vi "Configure Measurement (Power Meter).vi"(0 "VISA resource name":refnum<visa-resource-name>, 1 "Video Bandwidth Type (0: High)":i32(ring) items=["High", "Medium", "Low", "Off"], 2 "Gate Start Time (0 seconds)":dbl, 5 "Auto Power Range Enable (T: Enable)":bool=TRUE, 7 "Power Range (0: Upper)":i32(ring) items=["Upper", "Lower"], 9 "Center Frequency (1000 Hz)":dbl=1000.0, 11 "error in (no error)":errorcluster, 12 "Interval Time (0.1 seconds)":dbl=0.1, 13 "Gate Measurement Type (0: Peak)":i32(ring) items=["Peak", "Peak to Average", "Average", "Minimum"]) -> (4 "VISA resource name out":refnum<visa-resource-name>, 15 "error out":errorcluster)   [LabVIEW 2022 SP3, in "Agilent N934X Series.lvlib"]
doc: "Configures the cable setting of Power Meter Option.\n\nNotes:\n(1) Option PWM or PWP is required to enable this function. Option PWM supports Keysight (Agilent) U2000 series USB average power sensor, and Option PWP supports Keysight (Agilent) U2020 X series peak power sensor.\n\n(2) This VI is only applicable for N9321C, N9322C, N9323C, N9324C models"
uses:
  <instrlib>/Agilent N934X Series/Agilent N934X Series.lvlib
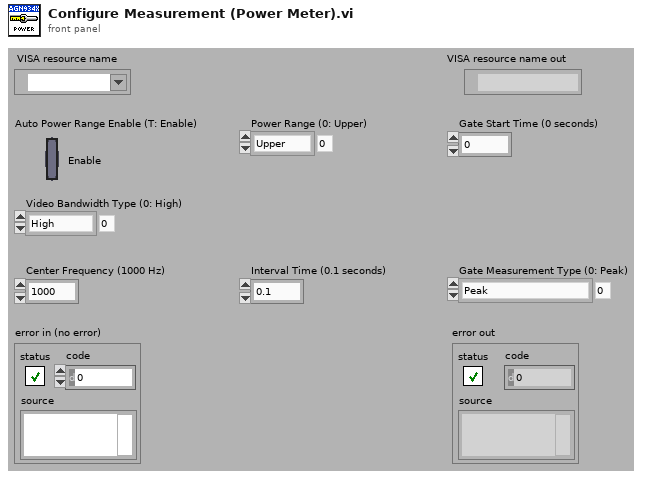
[diagram p1: front panel]
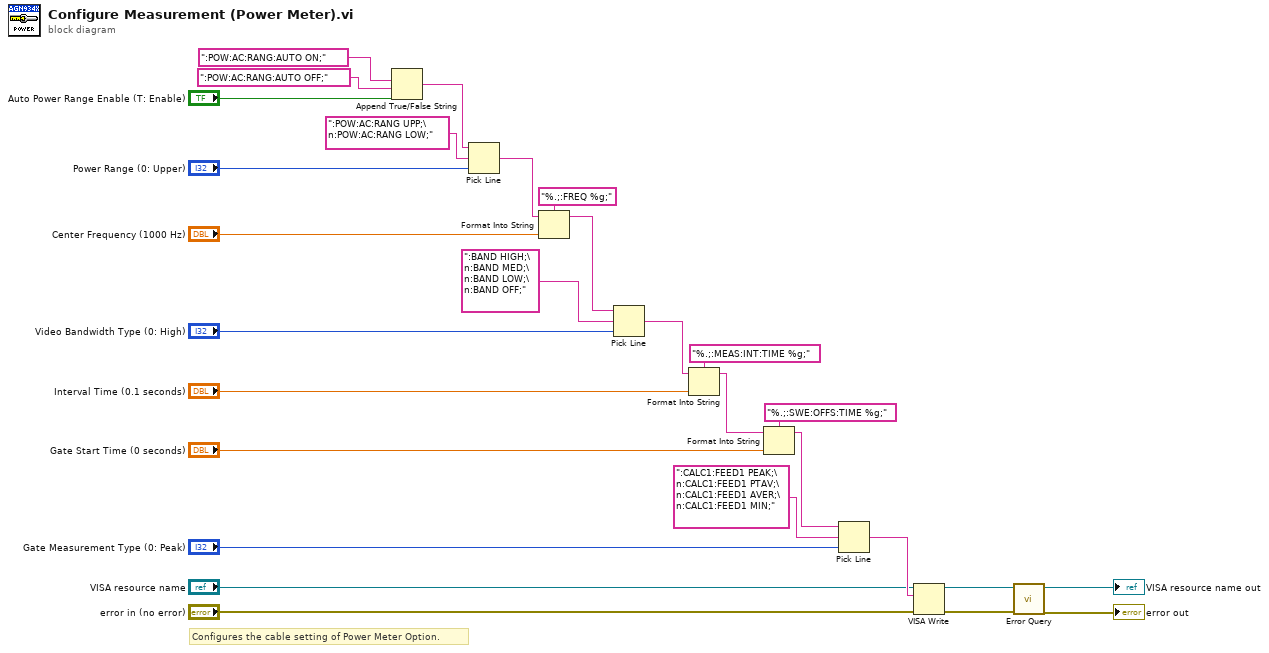
[diagram p0: block diagram]
diagram:
  # "Configures the cable setting of Power Meter Option."
  n1 = Append True/False String(1:"Auto Power Range Enable (T: Enable)", 2:":POW:AC:RANG:AUTO OFF;", 3:":POW:AC:RANG:AUTO ON;") -> (0:w1:string)  [unwired: 1 in]
  n2 = Pick Line(string ("")=w1, multi-line string=":POW:AC:RANG UPP;\n:POW:AC:RANG LOW;", line index="Power Range (0: Upper)") -> (output string=w2:string)
  n3 = Format Into String(format string="%.;:FREQ %g;", initial string=w2, "Center Frequency (1000 Hz)") -> (resulting string=w19:string)  [unwired: 1 in, 1 out]
  n4 = Pick Line(string ("")=w19, multi-line string=":BAND HIGH;\n:BAND MED;\n:BAND LOW;\n:BAND OFF;", line index="Video Bandwidth Type (0: High)") -> (output string=w18:string)
  n5 = Format Into String(format string="%.;:MEAS:INT:TIME %g;", initial string=w18, "Interval Time (0.1 seconds)") -> (resulting string=w15:string)  [unwired: 1 in, 1 out]
  n6 = Format Into String(format string="%.;:SWE:OFFS:TIME %g;", initial string=w15, "Gate Start Time (0 seconds)") -> (resulting string=w10:string)  [unwired: 1 in, 1 out]
  n7 = Pick Line(string ("")=w10, multi-line string=":CALC1:FEED1 PEAK;\n:CALC1:FEED1 PTAV;\n:CALC1:FEED1 AVER;\n:CALC1:FEED1 MIN;", line index="Gate Measurement Type (0: Peak)") -> (output string=w9:string)
  n8 = VISA Write(VISA resource name="VISA resource name", write buffer=w9, error in (no error)="error in (no error)") -> (VISA resource name out=w6:refnum<visa-resource-name>, error out=w5:errorcluster)  [unwired: 1 out]
  n9 = call <instrlib>:"Error Query.vi"("error in (no error)"=w5, "VISA resource name"=w6) -> ("error out"=→"error out":errorcluster, "VISA resource name out"=→"VISA resource name out":refnum<visa-resource-name>)  [unwired: 6 in, 2 out]
